vi "CNR project parameters.vi"(7 "bounds":T1, 8 "error in":errorcluster, 11 "parameters":dbl[](array[numeric])) -> (0 "error out":errorcluster, 3 "projected parameters":dbl[](array[numeric]))   [LabVIEW 2024, in "NI_Gmath.lvlib"]
uses:
  NI_Gmath.lvlib
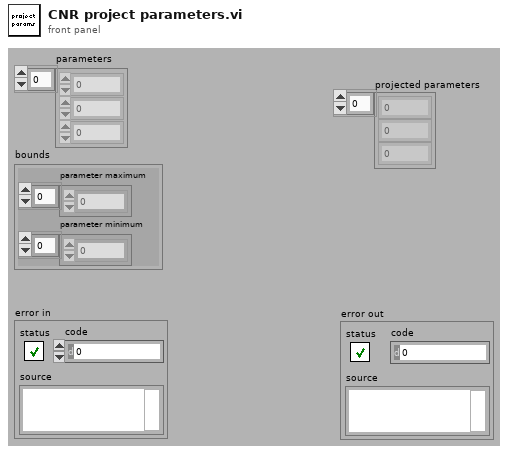
[diagram p1: front panel]
types:
  T1 = cluster{"parameter minimum":dbl[], "parameter maximum":dbl[]}
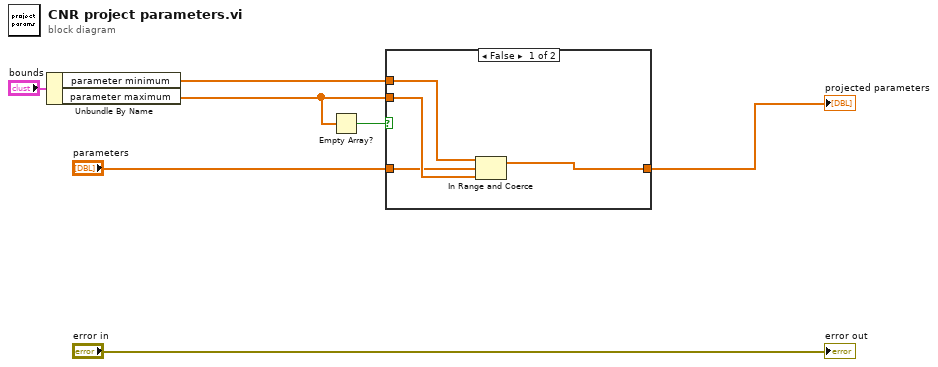
[diagram p0: block diagram]
diagram:
  n1 = Unbundle By Name("bounds") -> ("parameter minimum"=w3:dbl[], "parameter maximum"=w2:dbl[])
  n2 = Empty Array?(array=w2) -> (empty?=w1:bool)
  n3 = case shown="False" w1 {
    tunnel: [w11 w12] -> w5
    tunnel: w3 -> [w10 _]
    tunnel: w2 -> [w9 _]
    tunnel: "parameters" -> [w8 w12]
    frame False {
      n4 = In Range and Coerce(upper limit=w10, x=w8, lower limit=w9) -> (coerced(x)=w11:dbl[])  [unwired: 1 out]
    }
    frame True {
    }
  }
  "projected parameters" <- w5
  "error out" <- "error in"
